vi "ModifyStepSetup.vi"(8 "error in (no error)":errorcluster, 11 "Project.lvclass In":refnum<class "Project.lvclass">) -> (0 "error out":errorcluster, 3 "Project.lvclass Out":refnum<class "Project.lvclass">)   [LabVIEW 2014, in "Project.lvclass"]
uses:
  Project.lvclass
  StepSetupDataTypeDefine.ctl
  StepData/Control/AllStepTypeData.ctl
  StepData/Control/StepTypeEnum.ctl
  StepData/Control/MoveData.ctl
  StepData/Control/MeasureData.ctl
  Project.lvclass/Project.ctl
  AbstractStep/AbstractStep.lvclass
  StepData/StepData.lvclass
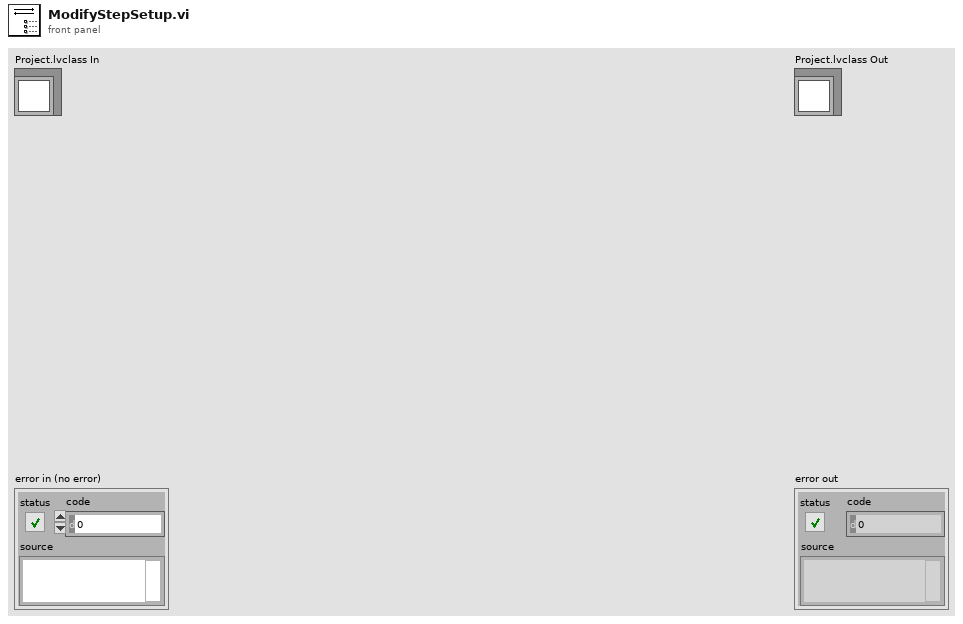
[diagram p1: front panel]
types:
  T1 = typedef "Project.lvclass/StepSetupDataTypeDefine.ctl" = cluster{"AllStepTypeData":T2}[]
  T2 = typedef "StepData.lvclass/AllStepTypeData.ctl" = cluster{"StepName":string, "StepTypeEnum":T3, "MoveData":T4, "MeasureData":T5}
  T3 = typedef "StepData.lvclass/StepTypeEnum.ctl" = enum16{"Move", "Measure"}
  T4 = typedef "StepData.lvclass/MoveData.ctl" = cluster{"Axis":u16, "Position":dbl, "Speed":dbl, "Acc/Dec":dbl, "Mode":u16}
  T5 = typedef "StepData.lvclass/MeasureData.ctl" = cluster{"Sensor No.":i32, "Log?":bool}
  T6 = typedef "Project.lvclass/ProjectDataTableTypeDefine.ctl" = string[][]
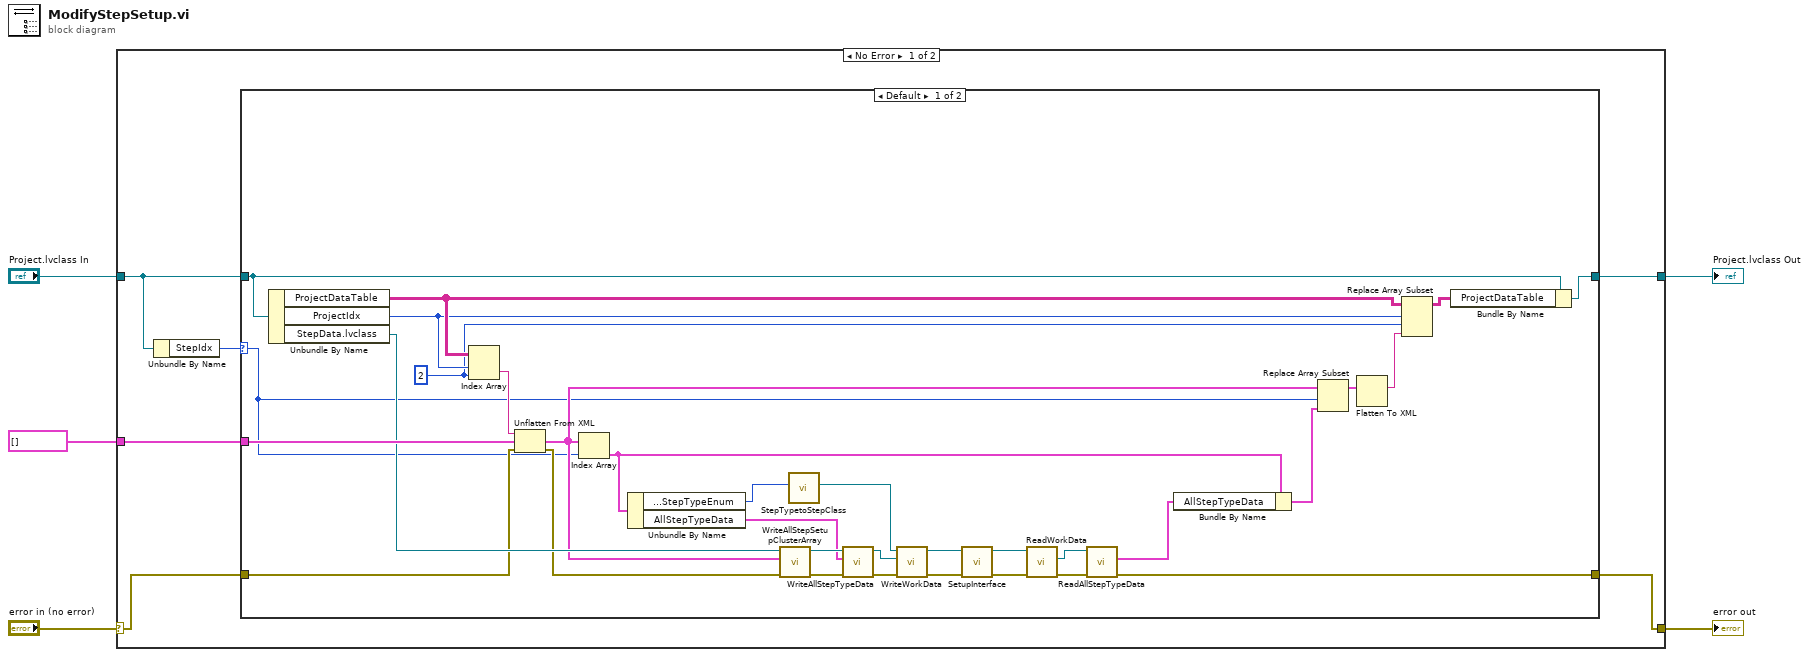
[diagram p0: block diagram]
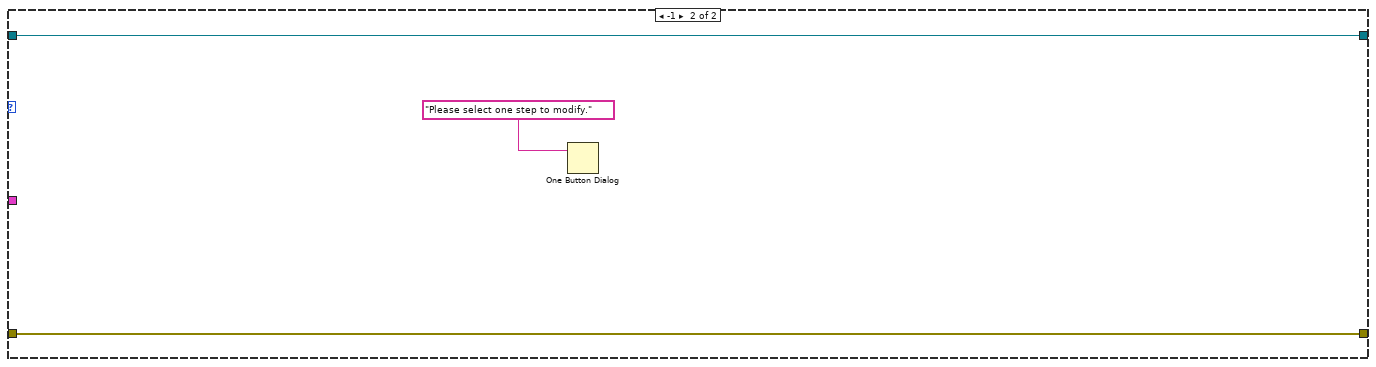
[diagram p2: hidden frame]
diagram:
  n1 = case shown="No Error" "error in (no error)" {
    selector: "error in (no error)" -> [w7 w48]
    tunnel: [w6 w48] -> w4
    tunnel: "Project.lvclass In" -> [w10 w47]
    tunnel: [w9 w47] -> w2
    tunnel: T1 [] ("StepSetupClusterArray") -> [w8 _]
    frame No Error {
      n2 = Unbundle By Name(w10) -> ("StepIdx"=w11:i32)
      n3 = case shown="Default" w11 {
        selector: w11 -> [w12 _]
        tunnel: w10 -> [w43 w46]
        tunnel: [w42 w46] -> w9
        tunnel: w8 -> [w40 _]
        tunnel: w7 -> [w13 w45]
        tunnel: [w14 w45] -> w6
        frame Default {
          w33 = 2 ("disabled index (col)")
          n4 = Unbundle By Name(w43) -> ("ProjectDataTable"=w36:T6, "ProjectIdx"=w34:i32, "StepData.lvclass"=w31:refnum<class "StepData.lvclass">)
          n5 = Index Array(array=w36, index (row)=w34, index (col)=w33) -> (element=w41:string)
          n6 = Unflatten From XML(xml string=w41, type=w40, error in (no error)=w13) -> (value=w30:T1, error out=w28:errorcluster)
          n7 = Index Array(array=w30, index=w12) -> (element=w39:cluster{"AllStepTypeData":T2})
          n8 = Unbundle By Name(w39) -> ("AllStepTypeData.StepTypeEnum"=w25:T3, "AllStepTypeData"=w26:T2)
          n9 = call "WriteAllStepSetupClusterArray.vi"("error in (no error)"=w28, "AllStepSetupClusterArray"=w30, "StepData.lvclass In"=w31) -> ("error out"=w27:errorcluster, "StepData.lvclass Out"=w29:refnum<class "StepData.lvclass">)  [unwired: 7 in]
          n10 = call "StepTypetoStepClass.vi"("StepTypeEnum"=w25) -> ("AbstractStep out"=w24:refnum<class "AbstractStep.lvclass">)  [unwired: 10 in]
          n11 = call "WriteAllStepTypeData.vi"("error in (no error)"=w27, "AllStepTypeData"=w26, "StepData.lvclass In"=w29) -> ("error out"=w22:errorcluster, "StepData.lvclass Out"=w23:refnum<class "StepData.lvclass">)  [unwired: 7 in]
          n12 = call-dynamic "WriteWorkData.vi"("error in (no error)"=w22, "StepData.lvclass"=w23, "AbstractStep in"=w24) -> ("error out"=w20:errorcluster, "AbstractStep out"=w21:refnum<class "AbstractStep.lvclass">)  [unwired: 7 in]
          n13 = call-dynamic "SetupInterface.vi"("error in (no error)"=w20, "AbstractStep in"=w21) -> ("error out"=w18:errorcluster, "AbstractStep out"=w19:refnum<class "AbstractStep.lvclass">)  [unwired: 8 in]
          n14 = call-dynamic "ReadWorkData.vi"("error in (no error)"=w18, "AbstractStep in"=w19) -> ("error out"=w17:errorcluster, "StepData.lvclass"=w16:refnum<class "StepData.lvclass">)  [unwired: 7 in, 1 out]
          n15 = call "ReadAllStepTypeData.vi"("error in (no error)"=w17, "StepData.lvclass In"=w16) -> ("error out"=w14:errorcluster, "AllStepTypeData"=w15:T2)  [unwired: 7 in, 1 out]
          n16 = Bundle By Name(cluster=w39, "AllStepTypeData"=w15) -> (w38:cluster{"AllStepTypeData":T2})
          n17 = Replace Array Subset(array=w30, new element=w38, index=w12) -> (w37:T1)
          n18 = Flatten To XML(anything=w37) -> (xml string=w32:string)
          n19 = Replace Array Subset(array=w36, new element=w32, index (row)=w34, index (col)=w33) -> (w35:T6)
          n20 = Bundle By Name(cluster=w43, "ProjectDataTable"=w35) -> (w42:refnum<class "Project.lvclass">)
        }
        frame -1 {
          n21 = One Button Dialog(message="Please select one step to modify.") -> ()  [unwired: 1 in, 1 out]
        }
      }
    }
    frame Error {
    }
  }
  "error out" <- w4
  "Project.lvclass Out" <- w2
